vi "Split Wavefrom Subsets.vi"(8 "error in (no error)":errorcluster, 9 "Waveforms in":waveform(dbl)[](array[waveform]), 11 "WaveformGraph in":refnum<vi>) -> (0 "error out":errorcluster, 1 "Waveform Subsets":waveform(dbl)[](array[waveform]), 2 "Waveform Subset 2":waveform(dbl), 3 "Waveform Subset 1":waveform(dbl))   [LabVIEW 2017]
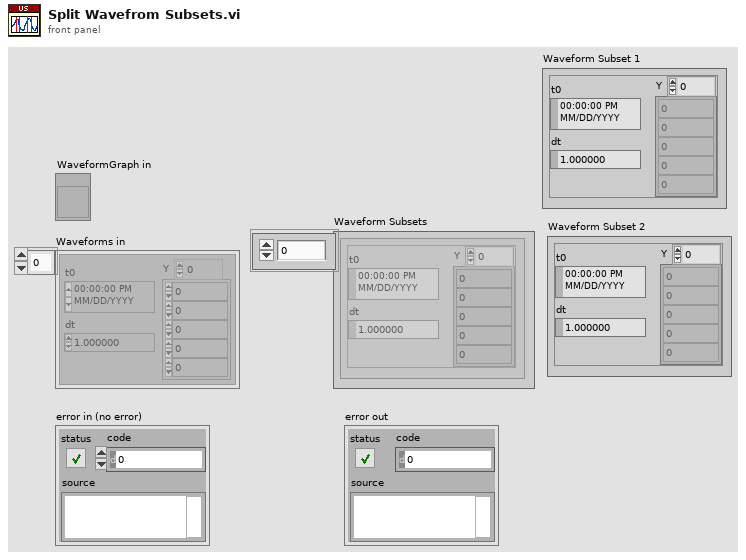
[diagram p1: front panel]
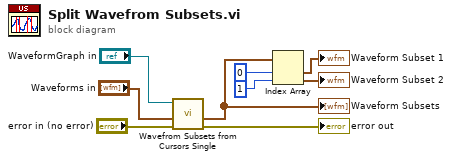
[diagram p0: block diagram]
diagram:
  n1 = call "Wavefrom Subsets from Cursors Single.vi"("Error In"="error in (no error)", "Waveforms In"="Waveforms in", "Waveform Graph"="WaveformGraph in") -> ("Error Out"=→"error out":errorcluster, "Waveform Subsets"=w5:waveform(dbl)[])  [unwired: 7 in]
  "Waveform Subsets" <- w5
  n2 = Index Array(array=w5, index #1=0 ("index (row)"), index #2=1 ("disabled index (col)")) -> (element #1=→"Waveform Subset 1":waveform(dbl), element #2=→"Waveform Subset 2":waveform(dbl))
